vi "Init_Instr.vi"(8 "error in (no error)":errorcluster caption="entrée d'erreur (pas d'erreur)", 11 "Class Instrument Firebase Altyor en entrée":refnum<class "Class Instrument Database Altyor.lvclass">) -> (0 "error out":errorcluster caption="sortie d'erreur", 3 "Class Instrument Firebase Altyor en sortie":refnum<class "Class Instrument Database Altyor.lvclass">)   [LabVIEW 2020, in "Library Instrument & Equipement.lvlib" / "Library Instruments.lvlib" / "Class Instrument Database Altyor.lvclass"]
uses:
  Class Instrument Database Altyor.lvclass
  Class Instrument Database Altyor.lvclass/Class Instrument Database Altyor.ctl
  Database/Database Altyor/Database Altyor.lvclass
  C:/Users/ngarcin/OneDrive - Altyor/Standard TB/Class/Database/Database drivers/Database Drivers.lvclass
  Instrument (Default)/Class Instrument (Default).lvclass
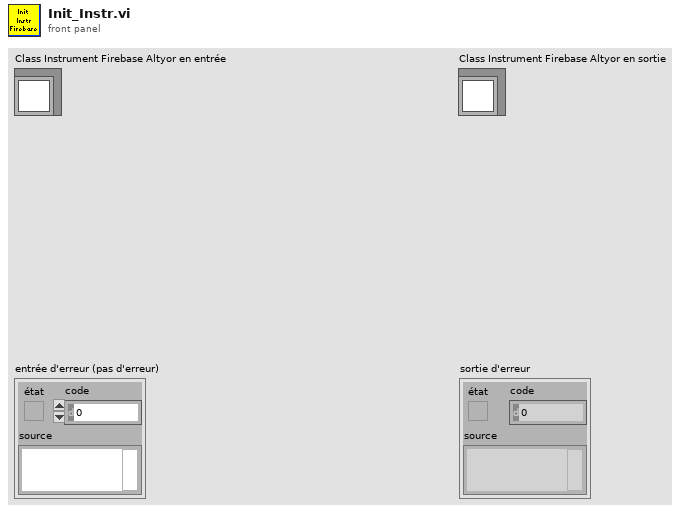
[diagram p1: front panel]
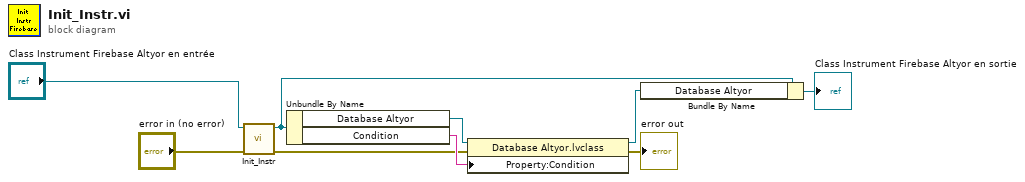
[diagram p0: block diagram]
diagram:
  n1 = call-parent "Init_Instr.vi"("error in (no error)"="error in (no error)", "Class Instrument (Default) en entrée"="Class Instrument Firebase Altyor en entrée") -> ("error out"=w2:errorcluster, "Class Instrument (Default) en sortie"=w5:refnum<class "Class Instrument Database Altyor.lvclass">)  [unwired: 8 in]
  n2 = Unbundle By Name(w5) -> ("Database Altyor"=w1:refnum<class "Database Altyor.lvclass">, "Condition"=w7:string)
  n3 = property class="Database Altyor.lvclass"(reference=w1, error in=w2, "Property:Condition"=w7) -> (reference out=w6:refnum<class "Database Altyor.lvclass">, error out=→"error out":errorcluster)
  n4 = Bundle By Name(cluster=w5, "Database Altyor"=w6) -> (→"Class Instrument Firebase Altyor en sortie":refnum<class "Class Instrument Database Altyor.lvclass">)
